vi "IMS Stepper Read Velocity.vi"(4 "error in (no error)":errorcluster, 7 "Instrument Address":refnum<visa-resource-name>) -> (0 "error out":errorcluster, 2 "Velocity":i32, 3 "dup VISA Resource Name":refnum<visa-resource-name>)   [LabVIEW 2025]
doc: "Author: Scott Hannahs <sth@magnet.fsu.edu>\n\nThis software is licensed for use under the “MIT License\"\nCopyright (c) 2025 Scott Hannahs, sth@sth@magnet.sthnet.net\n\nPermission is hereby granted, free of charge, to any person obtaining a copy of this software and associated documentation files (the \"Software\"), to deal in the Software without restriction, including without limitation the rights to use, copy, modify, merge, publish, distribute, sublicense, and/or sell copies of the Software, and to permit persons to whom the Software is furnished to do so, subject to the following conditions: The above copyright notice and this permission notice shall be included in all copies or substantial portions of the Software.\n\nTHE SOFTWARE IS PROVIDED \"AS IS\", WITHOUT WARRANTY OF ANY KIND, EXPRESS OR IMPLIED, INCLUDING BUT NOT LIMITED TO THE WARRANTIES OF MERCHANTABILITY, FITNESS FOR A PARTICULAR PURPOSE AND NONINFRINGEMENT. IN NO EVENT SHALL THE AUTHORS OR COPYRIGHT HOLDERS BE LIABLE FOR ANY CLAIM, DAMAGES OR OTHER LIABILITY, WHETHER IN AN ACTION OF CONTRACT, TORT OR OTHERWISE, ARISING FROM, OUT OF OR IN CONNECTION WITH THE SOFTWARE OR THE USE OR OTHER DEALINGS IN THE SOFTWARE."
uses:
  <vilib>/regexp/Match Regular Expression.xnode
panel:
  out "Response":string
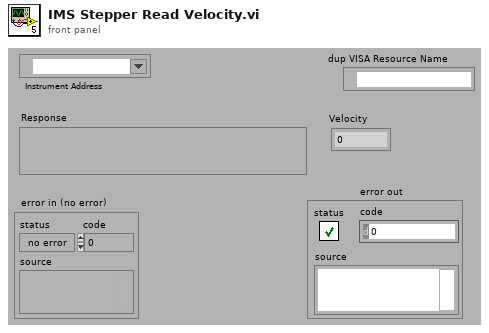
[diagram p1: front panel]
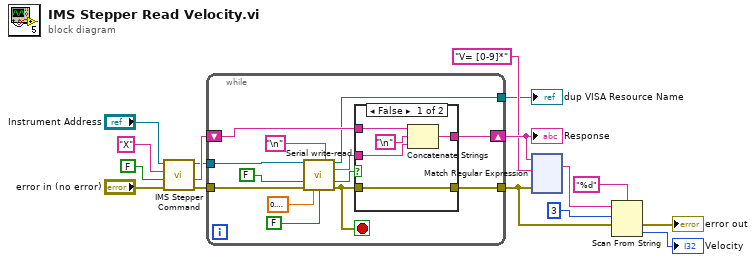
[diagram p0: block diagram]
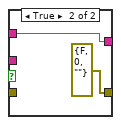
[diagram p2: hidden frame]
diagram:
  n1 = call "IMS Stepper Command.vi"("error in (no error)"="error in (no error)", "Mode"=FALSE, "Command"="X", "Instrument Address"="Instrument Address") -> ("error out"=w16:errorcluster, "Response"=w15:string, "Instrument Address Out"=w1:refnum<visa-resource-name>)  [unwired: 2 in, 1 out]
  n2 = while {
    tunnel: w1 -> [w29]
    tunnel: w16 -> [w28]
    shift-right: [w21] -> w14
    shift-left: w15 -> [w23]
    tunnel: [w18] -> w3
    tunnel: [w19] -> w4
    stop <- w17 stop-if-true
    n3 = call "Serial write-read.vi"("VISA Resource Name"=w29, "EOT Chars (cr/lf)"="\n", "Clear Buffer?"=FALSE, "error in (no error)"=w28, "Timeout Limit"=sgl 0.1, "Read Echo?"=FALSE) -> ("dup VISA Resource Name"=w19:refnum<visa-resource-name>, "Serial Read"=w22:string, "Timeout"=w20:bool, "error out"=w17:errorcluster)  [unwired: 4 in, 2 out]
    n4 = case shown="False" w20 {
      tunnel: w23 -> [w34 w36]
      tunnel: w22 -> [w32 _]
      tunnel: [w33 w36] -> w21
      tunnel: [w30 errorcluster {"status"=FALSE, "code"=0, "source"=""} ("error out")] -> w18
      tunnel: w17 -> [w30 _]
      frame False {
        n5 = Concatenate Strings(w34, "\n", w32) -> (w33:string)
      }
      frame True {
      }
    }
  }
  "Response" <- w14
  "dup VISA Resource Name" <- w4
  n6 = xnode "Match Regular Expression"("input string"=w14, "regular expression"="V= [0-9]*", "error in"=w3) -> ("whole match"=w12:string)  [unwired: 3 in, 4 out]
  n7 = Scan From String(format string="%d", input string=w12, initial scan location=u32 3, error in=w3) -> (error out=→"error out":errorcluster, output 1=→"Velocity":i32)  [unwired: 1 in, 2 out]
